vi "2. Set Label Position.vi"(6 "Variant in":variant, 7 "Shift Pressed?":bool, 8 "error in (no error)":errorcluster, 10 "QD Combo Box Ref":refnum<vi>, 11 "QD Launch VI Ref":refnum<vi>) -> (0 "error out":errorcluster, 4 "Variant out":variant)   [LabVIEW 2010]
doc: "Default Shortcut - [2]"
uses:
  <vilib>/Utility/config.llb/NI_LVConfig.lvlib
  <vilib>/Utility/config.llb/Read Key (String).vi
panel:
  in  "Undo Name":string="Quick Drop Keyboard Shortcut"
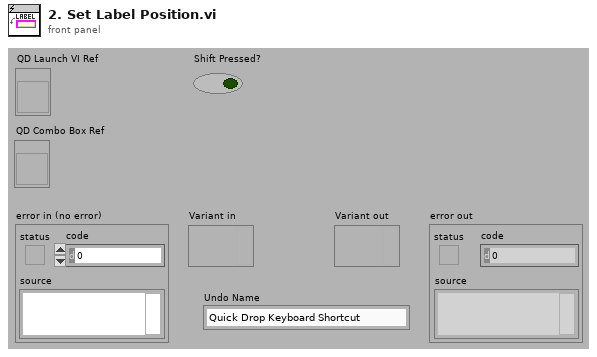
[diagram p1: front panel]
types:
  T1 = typedef "NI_LVConfig.lvlib/Config Data RefNum.ctl" = refnum<k1>
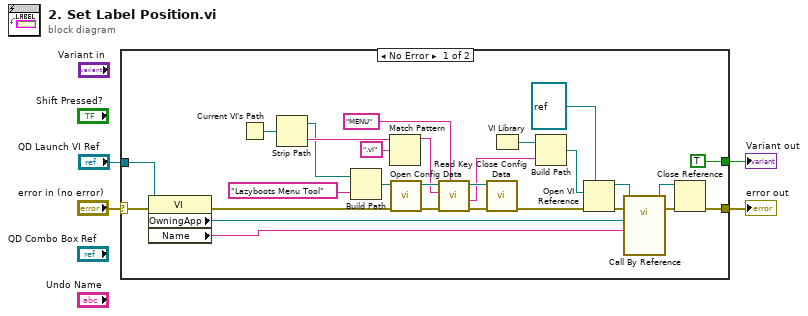
[diagram p0: block diagram]
diagram:
  n1 = case shown="No Error" "error in (no error)" {
    selector: "error in (no error)" -> [w32 w33]
    tunnel: [w31 w33] -> w3
    tunnel: "QD Launch VI Ref" -> [w30 _]
    tunnel: [TRUE _] -> w1
    frame No Error {
      n2 = property class="VI"(reference=w30, error in=w32) -> (error out=w10:errorcluster, "OwningApp"=w12:refnum<vi>, "Name"=w11:string)  [unwired: 1 out]
      n3 = Current VI's Path() -> (path=w26:path)
      n4 = Strip Path(path=w26) -> (stripped path=w8:path, name=w18:string)
      n5 = Build Path(base path=w8, name or relative path="Lazyboots Menu Tool") -> (appended path=w24:path)
      n6 = Match Pattern(string=w18, regular expression=".vi") -> (before substring=w17:string)  [unwired: 4 out]
      n7 = call <vilib>:"Open Config Data.vi"("error in (no error)"=w10, "configuration file path"=w24) -> ("error out"=w22:errorcluster, "refnum"=w23:T1)  [unwired: 7 in, 1 out]
      n8 = call-poly <vilib>:"Read Key.vi"("section"="MENU", "error in (no error)"=w22, "key"=w17, "refnum"=w23) -> ("error out"=w19:errorcluster, "value"=w14:string, "refnum out"=w20:T1)  [unwired: 2 in, 3 out]
      n9 = call <vilib>:"Close Config Data.vi"("error in (no error)"=w19, "refnum"=w20) -> ("error out"=w9:errorcluster)  [unwired: 1 in, 8 out]
      n10 = VI Library() -> (path=w13:path)
      n11 = Build Path(base path=w13, name or relative path=w14) -> (appended path=w15:path)
      n12 = Open VI Reference(type specifier VI Refnum (for type only)=refnum<vi> refnum, vi path=w15, error in (no error)=w9) -> (vi reference=w6:refnum<vi>, error out=w28:errorcluster)  [unwired: 3 out]
      n13 = call-by-ref "?"(reference=w6, error in=w28, "VI Path"=w11, "Application Reference"=w12) -> (reference out=w7:refnum<vi>, error out=w27:errorcluster)  [unwired: 9 in, 1 out]
      n14 = Close Reference(reference=w7, error in (no error)=w27) -> (error out=w31:errorcluster)
    }
    frame Error {
    }
  }
  "error out" <- w3
  "Variant out" <- w1
